vi "MarkPlayerPosition.vi"(7 "Player":enum16{"Player1", "Player2"}(ring), 8 "error in (no error)":errorcluster, 10 "NewPosition":T1, 11 "Board in":refnum<class "Board.lvclass">) -> (0 "error out":errorcluster, 2 "AlreadyOccupied":bool, 3 "Board out":refnum<class "Board.lvclass">)   [LabVIEW 2015, in "TronviewGame.lvlib" / "Board.lvclass"]
uses:
  Board.lvclass
  Position.ctl
  BoardSize.ctl
  FieldState.ctl
  Board.lvclass/Board.ctl
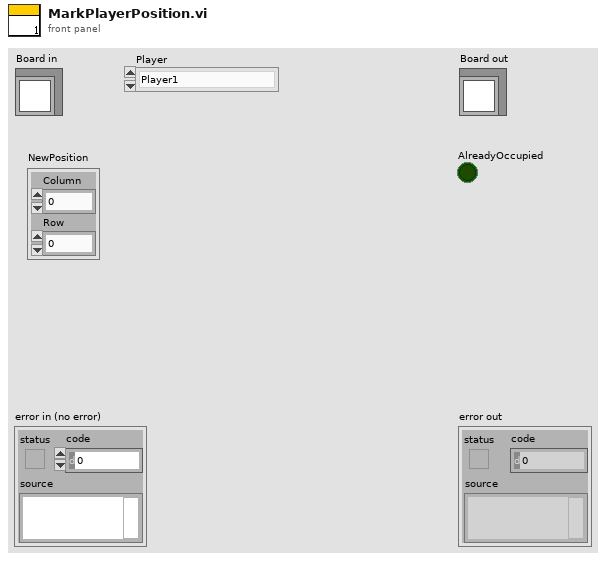
[diagram p1: front panel]
types:
  T1 = typedef "TronviewGame.lvlib/Board.lvclass/Position.ctl" = cluster{"Column":i32, "Row":i32}
  T2 = typedef "TronviewGame.lvlib/Board.lvclass/BoardSize.ctl" = cluster{"Columns":u32, "Rows":u32}
  T3 = typedef "TronviewGame.lvlib/Board.lvclass/FieldState.ctl" = enum16{"Empty", "Blocked", "Player1Position", "Player2Postion", "Player1Marked", "Player2Marked"}
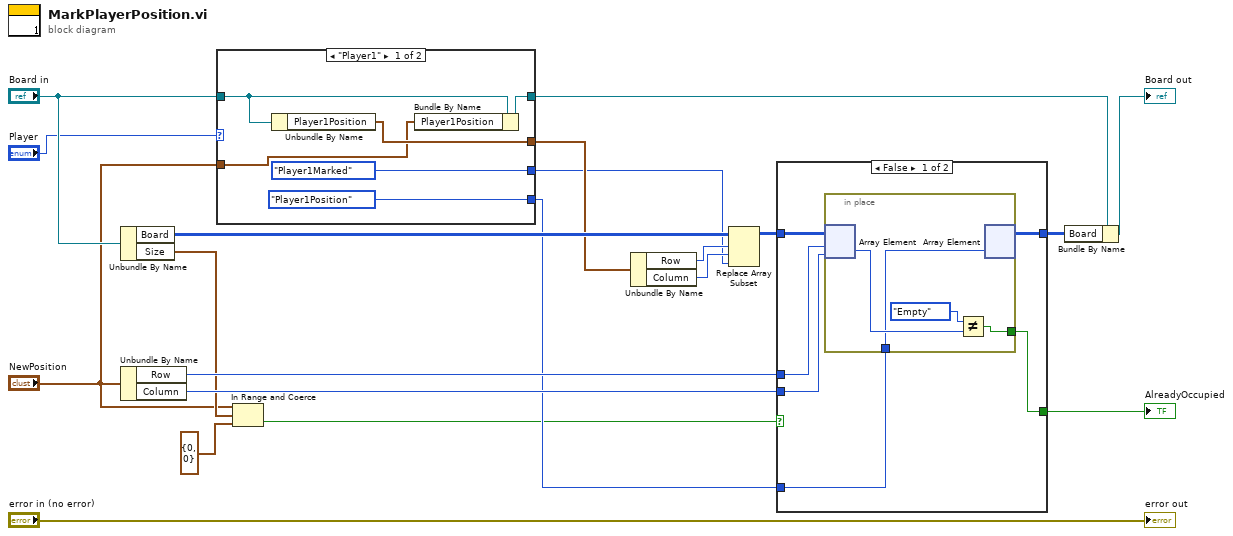
[diagram p0: block diagram]
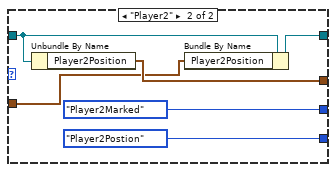
[diagram p2: hidden frame]
diagram:
  n1 = Unbundle By Name("Board in") -> ("Board"=w14:T3[][], "Size"=w7:T2)
  n2 = Unbundle By Name("NewPosition") -> ("Row"=w19:i32, "Column"=w18:i32)
  n3 = case shown="\"Player1\"" "Player" {
    tunnel: [FieldState."Player1Marked" ("element") FieldState."Player2Marked" ("element")] -> w8
    tunnel: [FieldState."Player1Position" ("element") FieldState."Player2Postion" ("element")] -> w12
    tunnel: [w23 w29] -> w11
    tunnel: "Board in" -> [w24 w30]
    tunnel: [w22 w28] -> w3
    tunnel: "NewPosition" -> [w21 w27]
    frame "Player1" {
      n4 = Unbundle By Name(w24) -> ("Player1Position"=w23:T1)
      n5 = Bundle By Name(cluster=w24, "Player1Position"=w21) -> (w22:refnum<class "Board.lvclass">)
    }
    frame "Player2" {
      n6 = Unbundle By Name(w30) -> ("Player2Position"=w29:T1)
      n7 = Bundle By Name(cluster=w30, "Player2Position"=w27) -> (w28:refnum<class "Board.lvclass">)
    }
  }
  n8 = In Range and Coerce(upper limit="NewPosition", x=w7, lower limit=T2 {"Columns"=0, "Rows"=0}) -> (In Range?=w5:bool)  [unwired: 1 out]
  n9 = Unbundle By Name(w11) -> ("Row"=w10:i32, "Column"=w9:i32)
  n10 = Replace Array Subset(array=w14, new element=w8, index (row)=w10, index (col)=w9) -> (w13:T3[][])
  n11 = case shown="False" w5 {
    selector: w5 -> [_ w43]
    tunnel: w13 -> [w34 w44]
    tunnel: w19 -> [w38 _]
    tunnel: w18 -> [w37 _]
    tunnel: [w36 w43] -> w15
    tunnel: [w35 w44] -> w16
    tunnel: w12 -> [w33 _]
    frame False {
      n12 = in-place {
        in-place-border: [w40] -> w36
        in-place-border: w33 -> [w39]
        n13 = in-place-array #1(w34, w38, w37) -> (w42:T3)
        n14 = Not Equal?(x=FieldState."Empty", y=w42) -> (x != y?=w40:bool)
        n15 = in-place-array #1(w39) -> (w35:T3[][])  [unwired: 2 out]
      }
    }
    frame True {
    }
  }
  "AlreadyOccupied" <- w15
  n16 = Bundle By Name(cluster=w3, "Board"=w16) -> (→"Board out":refnum<class "Board.lvclass">)
  "error out" <- "error in (no error)"
